vi "WPI_MotorControlTrackCANSemaphores.vi"(8 "error in (no error)":errorcluster, 10 "Operation":T2(ring), 11 "semaphore":T1) -> (0 "error out":errorcluster)   [LabVIEW 2025]
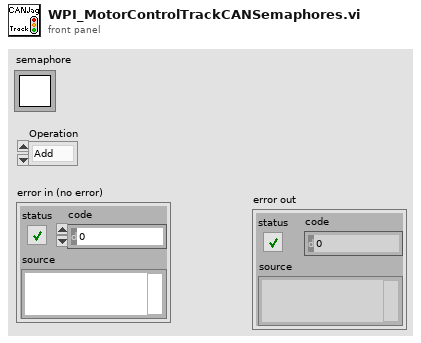
[diagram p1: front panel]
types:
  T1 = typedef "Semaphore RefNum" = refnum<k1>
  T2 = enum16{"Add", "Remove", "Acquire All", "Release All"}
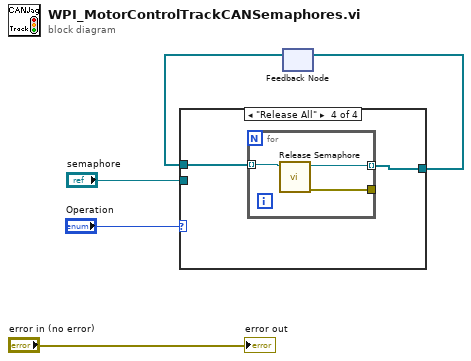
[diagram p0: block diagram]
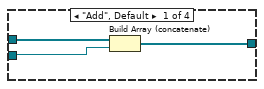
[diagram p2: hidden frame]
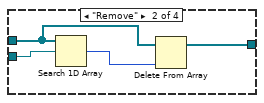
[diagram p3: hidden frame]
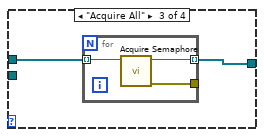
[diagram p4: hidden frame]
diagram:
  n1 = feedback #1() -> (w3:T1[])  [unwired: 1 in]
  n2 = case shown="\"Release All\"" "Operation" {
    tunnel: "semaphore" -> [w8 w12 _ _]
    tunnel: w3 -> [w7 w10 w14 w19]
    tunnel: [w6 w9 w13 w18] -> w2
    frame "Add", Default {
      n3 = Build Array (concatenate)(w7, w8) -> (w6:T1[])
    }
    frame "Remove" {
      n4 = Search 1D Array(1D array=w10, element=w12) -> (index of element=w11:i32)  [unwired: 1 in]
      n5 = Delete From Array(array=w10, index=w11) -> (array with subset deleted=w9:T1[])  [unwired: 1 in, 1 out]
    }
    frame "Acquire All" {
      n6 = for {
        tunnel: w14 -> [w17] mode=indexing
        tunnel: [w16] -> w13 mode=indexing
        tunnel: [w15] -> _
        n7 = call <vilib>:"Acquire Semaphore.vi"("semaphore"=w17) -> ("error out"=w15:errorcluster, "semaphore out"=w16:T1)  [unwired: 2 in, 3 out]
      }
    }
    frame "Release All" {
      n8 = for {
        tunnel: w19 -> [w22] mode=indexing
        tunnel: [w21] -> w18 mode=indexing
        tunnel: [w20] -> _
        n9 = call <vilib>:"Release Semaphore.vi"("semaphore"=w22) -> ("error out"=w20:errorcluster, "semaphore out"=w21:T1)  [unwired: 1 in, 4 out]
      }
    }
  }
  n10 = feedback-in #1(w2) -> ()
  "error out" <- "error in (no error)"
